vi "health_adam4022t_write_digital.vi"(5 "Address":string, 7 "Channel":string, 9 "Value":string, 11 "Error In":errorcluster) -> (8 "Response":string, 10 "Status":bool, 15 "Error Out":errorcluster)   [LabVIEW 2018]
doc: "The Basic Serial Read and Write example performs a Serial Port Read, a Serial Port Write, or a combination of these actions. The user selects the actions (read or write) on the front panel. If both are selected, the VI will write the data first, read data, and then close the VISA session that is opened to the port. This VI will wait until the specified number of bytes is received at the port. Only the number of bytes specified will be read.\n\nINSTRUCTIONS:\n1) Select the serial resource and configuration parameters (baud rate, data bits, parity, stop bits, flow control).\n2) Select the operations to be performed. \n3) Connect the serial port to your device. If no device is available, perform a loopback test by doing one of the following. Short pins 2 and 3 on a RS-232 cable or short pin 4 to pin 8 and pin 5 to pin 9 on a RS-485/422 cable. \n4) Run the VI to see the data read. (The \"read string\" will match the \"string to write\" if a loopback test was performed.)\n\nNote: The parameters set for the serial port must match the parameters of the connected instrument or device. In this example, the bytes to read parameter specifies the number of bytes that the serial port reads. If there were more bytes at the port than the number specified in bytes to read, those bytes would not be read. Also, if you specify to read more bytes than the number of bytes actually read, you might receive a timeout error message.\n\nOn the block diagram, the Configure Serial Port VI sets the configuration parameters. The front panel displays the controls used to configure the basic parameters, such as baud rate, data bits, and parity. Constants configure the other parameters the user probably does not need set. After the VISA Configure Serial Port VI opens the VISA session and configures the port, the VI passes the VISA resource name to other VIs that perform operations on that VISA resource. The VISA Write function sends a command to the serial device and the VISA Read function returns data based on the command. The VISA Close function then closes the reference to the serial device. It is important to close the reference; otherwise communication through with that port through protocols other than VISA might not be possible."
uses:
  <vilib>/Instr/_visa.llb/VISA Configure Serial Port (Instr).vi
panel:
  # "ADAM 4022T Serial Comm."
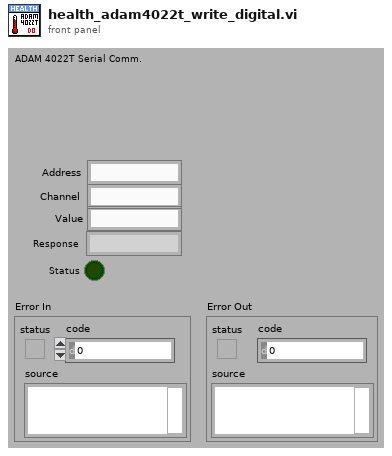
[diagram p1: front panel]
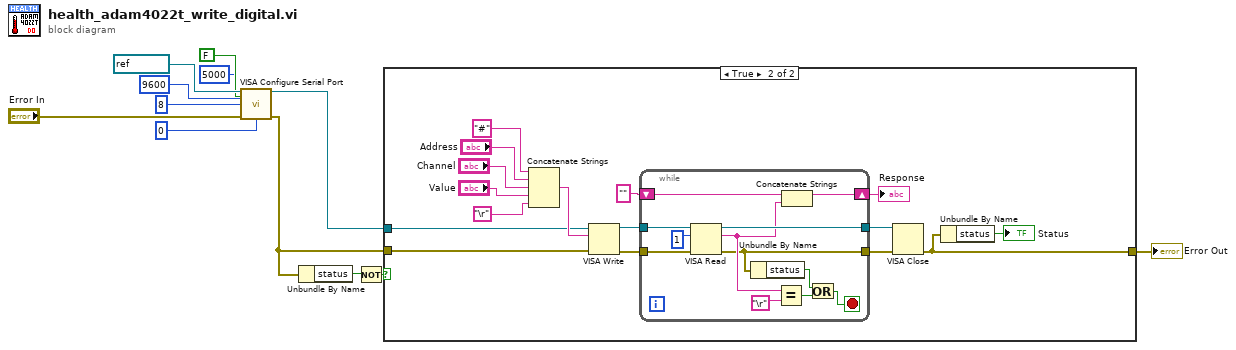
[diagram p0: block diagram]
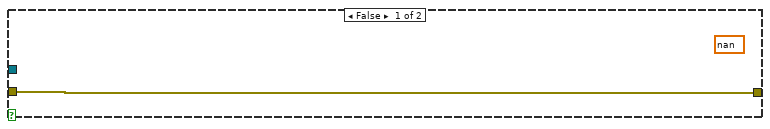
[diagram p2: hidden frame]
diagram:
  n1 = call-poly "VISA Configure Serial Port"("VISA resource name"=refnum<visa-resource-name> "Port1" ("adamSerial.port"), "timeout (10sec)"=u32 5000 ("adamSerial.timeout"), "Enable Termination\nChar (T)"=FALSE ("adamSerial.termChar"), "baud rate (9600)"=u32 9600 ("adamSerial.baud"), "data bits (8)"=u16 8 ("adamSerial.dataBits"), "error in (no error)"="Error In", "flow control (0:none)"=u16 0 ("adamSerial.flowControl")) -> ("VISA resource name out"=w12:refnum<visa-resource-name>, "error out"=w11:errorcluster)  [unwired: 7 in]
  n2 = Unbundle By Name(w11) -> ("status"=w9:bool)
  n3 = Not(x=w9) -> (.not. x?=w10:bool)
  n4 = case shown="True" w10 {
    tunnel: w12 -> [_ w26]
    tunnel: w11 -> [w13 w25]
    tunnel: [w13 w20] -> w8
    frame False {
      (unwired) nan ("t")
    }
    frame True {
      n5 = Concatenate Strings("#", "Address", "Channel", "Value", "\r") -> (w27:string)
      n6 = VISA Write(VISA resource name=w26, write buffer=w27, error in (no error)=w25) -> (VISA resource name out=w24:refnum<visa-resource-name>, error out=w23:errorcluster)  [unwired: 1 out]
      n7 = while {
        tunnel: [w30] -> w21
        tunnel: [w41] -> w29
        tunnel: w24 -> [w39]
        tunnel: w23 -> [w38]
        shift-right: [w35] -> w17
        shift-left: "" ("read buffer") -> [w36]
        stop <- w33 stop-if-true
        n8 = VISA Read(VISA resource name=w39, byte count=u32 1, error in (no error)=w38) -> (VISA resource name out=w41:refnum<visa-resource-name>, read buffer=w34:string, error out=w30:errorcluster)  [unwired: 1 out]
        n9 = Unbundle By Name(w30) -> ("status"=w31:bool)
        n10 = Equal?(x=w34, y="\r") -> (x = y?=w32:bool)
        n11 = Concatenate Strings(w36, w34) -> (w35:string)
        n12 = Or(x=w31, y=w32) -> (x .or. y?=w33:bool)
      }
      "Response" <- w17
      n13 = VISA Close(VISA resource name=w29, error in (no error)=w21) -> (error out=w20:errorcluster)
      n14 = Unbundle By Name(w20) -> ("status"=→"Status":bool)
    }
  }
  "Error Out" <- w8
